vi "Debug Exercise (Main).vi"() -> ()   [LabVIEW 2014]
doc: "This VI is an exercise in the LabVIEW Core I course.\n\nThis exercise is used to demonstrate the use of different debugging tools. First, fix the broken run arrow and then use the different debugging tools to see how they work."
panel:
  out "Final Result":dbl format="%.2f"
  out "Random Number":dbl format="%.2f"
  in  "Multiply Result":dbl format="%.2f"
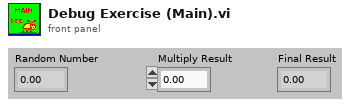
[diagram p1: front panel]
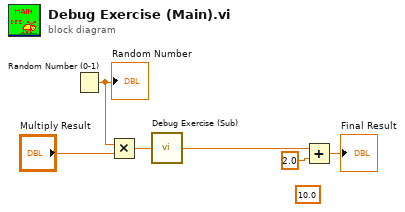
[diagram p0: block diagram]
diagram:
  (unwired) 10.0
  n1 = Random Number (0-1)() -> (number: 0 to 1=w6:dbl)
  "Random Number" <- w6
  n2 = Multiply(x=w6, y="Multiply Result") -> (x*y=w2:dbl)
  n3 = call "Debug Exercise (Sub).vi"("Number"=w2) -> ("Final Result"=w3:dbl)
  n4 = Add(x=w3, y=2.0) -> (x+y=→"Final Result":dbl)
